vi "xxxx Core.vi"(8 "error in (no error)":errorcluster, 11 "B Context State in":refnum<class "B Context State.lvclass">) -> (0 "error out":errorcluster, 3 "B Context State out":refnum<class "B Context State.lvclass">)   [LabVIEW 2021, in "Context Actor.lvlib" / "B Context State.lvclass"]
uses:
  B Context State.lvclass
  B Context State.lvclass/B Context State.ctl
  Context Actor.lvclass
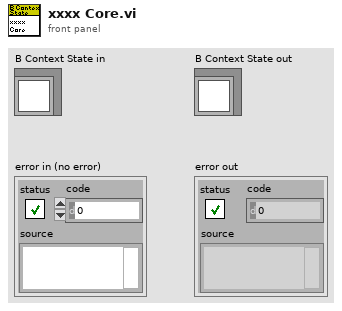
[diagram p1: front panel]
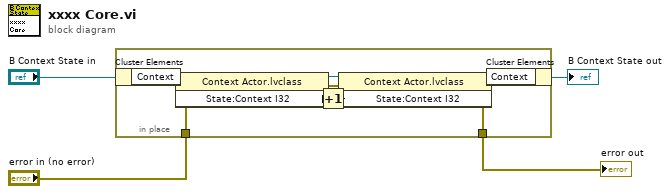
[diagram p0: block diagram]
diagram:
  n1 = in-place {
    in-place-border: "error in (no error)" -> [w7]
    in-place-border: [w5] -> w1
    n2 = in-place-cluster #1("B Context State in") -> ("Context"=w12:refnum<class "Context Actor.lvclass">)
    n3 = property class="Context Actor.lvclass"(reference=w12, error in=w7) -> (reference out=w11:refnum<class "Context Actor.lvclass">, error out=w6:errorcluster, "State:Context I32"=w9:i32)
    n4 = Increment(x=w9) -> (x+1=w8:i32)
    n5 = property class="Context Actor.lvclass"(reference=w11, error in=w6, "State:Context I32"=w8) -> (reference out=w10:refnum<class "Context Actor.lvclass">, error out=w5:errorcluster)
    n6 = in-place-cluster #1("Context"=w10) -> (→"B Context State out":refnum<class "B Context State.lvclass">)
  }
  "error out" <- w1
